vi "Point_Delete_Attribute.vi"(8 "Error In":errorcluster, 9 "Attribute":string, 10 "Tag":string, 11 "Map":T1) -> (0 "Error Out":errorcluster, 3 "Map Out":T1)   [LabVIEW 2017, in "PointValueMap.lvlib"]
uses:
  <vilib>/addons/PointValueMap/PointValueMap.lvlib
  <vilib>/addons/PointValueMap/controls/PointMap.ctl
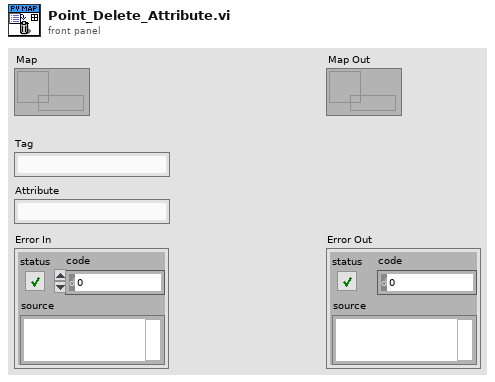
[diagram p1: front panel]
types:
  T1 = typedef "PointValueMap.lvlib/PointMap.ctl" = refnum<data-value>
  T2 = typedef "PointValueMap.lvlib/Point.ctl" = cluster{"Datatype":T3, "Timestamp":timestamp, "Value":variant, "Valid":bool}
  T3 = typedef "PointValueMap.lvlib/DataTypes.ctl" = enum16{"single", "double", "i32", "string", "variant"}
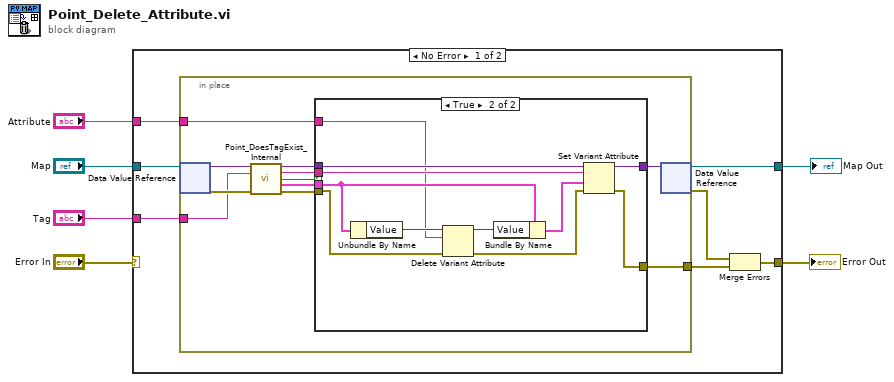
[diagram p0: block diagram]
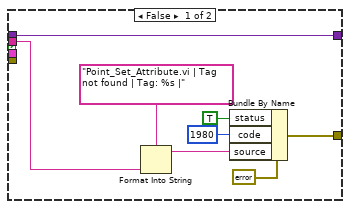
[diagram p2: hidden frame]
diagram:
  n1 = case shown="No Error" "Error In" {
    selector: "Error In" -> [_ w45]
    tunnel: "Map" -> [w13 w44]
    tunnel: "Tag" -> [w12 _]
    tunnel: [w10 w45] -> w5
    tunnel: [w9 w44] -> w1
    tunnel: "Attribute" -> [w8 _]
    frame No Error {
      n2 = in-place {
        in-place-border: w12 -> [w22]
        in-place-border: w8 -> [w16]
        in-place-border: [w14] -> w7
        n3 = in-place-dvr #1(w13) -> (w24:variant, w23:errorcluster)
        n4 = call <vilib>:"Point_DoesTagExist_Internal.vi"("Map"=w24, "Tag"=w22, "Error In"=w23) -> ("Map Out"=w21:variant, "Tag Out"=w20:string, "Tag Exists"=w19:bool, "Point"=w18:T2, "Error Out"=w17:errorcluster)  [unwired: 7 in, 1 out]
        n5 = case shown="True" w19 {
          tunnel: [w26 w43] -> w15
          tunnel: [w27 w42] -> w14
          tunnel: w16 -> [_ w35]
          tunnel: w21 -> [w26 w41]
          tunnel: w17 -> [_ w34]
          tunnel: w18 -> [_ w40]
          tunnel: w20 -> [w25 w38]
          frame False {
            n6 = Format Into String(format string="Point_Set_Attribute.vi | Tag not found | Tag: %s |" ("source"), w25) -> (resulting string=w29:string)  [unwired: 2 in, 1 out]
            n7 = Bundle By Name(cluster=errorcluster {"status"=FALSE, "code"=0, "source"=""} ("Error Out"), "status"=TRUE, "code"=1980, "source"=w29) -> (w27:errorcluster)
          }
          frame True {
            n8 = Unbundle By Name(w40) -> ("Value"=w37:variant)
            n9 = Delete Variant Attribute(4:w34, 6:w35, 7:w37) -> (0:w33:errorcluster, 3:w36:variant)  [unwired: 1 out]
            n10 = Bundle By Name(cluster=w40, "Value"=w36) -> (w39:T2)
            n11 = Set Variant Attribute(Variant=w41, name=w38, value=w39, error in=w33) -> (Variant out=w43:variant, error out=w42:errorcluster)  [unwired: 1 out]
          }
        }
        n12 = in-place-dvr #1(w15) -> (w9:T1, w11:errorcluster)
      }
      n13 = Merge Errors(w11, w7) -> (w10:errorcluster)
    }
    frame Error {
    }
  }
  "Error Out" <- w5
  "Map Out" <- w1
